vi "UniqueVals.vi"(10 "Array in":string[](array[string])) -> (2 "Unique List":string[](array[string]))   [LabVIEW 2013]
doc: "Make list of unique elements contained in Array in. To use for higher dimensions, flatten to 1D input."
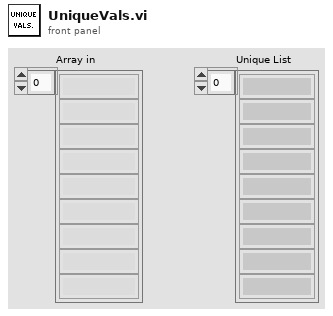
[diagram p1: front panel]
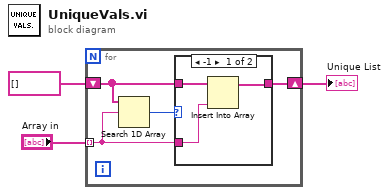
[diagram p0: block diagram]
diagram:
  n1 = for {
    tunnel: "Array in" -> [w4] mode=indexing
    shift-right: [w6] -> w1
    shift-left: string[] [] ("Unique List") -> [w7]
    n2 = Search 1D Array(1D array=w7, element=w4) -> (index of element=w5:i32)  [unwired: 1 in]
    n3 = case shown="-1" w5 {
      tunnel: w7 -> [w10 w11]
      tunnel: [w9 w11] -> w6
      tunnel: w4 -> [w8 _]
      frame -1 {
        n4 = Insert Into Array(array=w10, new element=w8) -> (w9:string[])  [unwired: 1 in]
      }
      frame Default {
      }
    }
  }
  "Unique List" <- w1
